vi "New Round.vi"(8 "error in (no error)":errorcluster, 10 "Move Count":i32, 11 "Grid in":T1) -> (0 "error out":errorcluster, 3 "Grid out":T1)   [LabVIEW 2015, in "TeamEffort.lvclass"]
uses:
  TeamEffort.lvclass
  Grid Cluster.ctl
  Player Cluster.ctl
  Square/Square.lvclass
  Team Move Input.ctl
  Type Defs/Action Enum.ctl
  Team Move Output.ctl
  Type Defs/Direction Enum.ctl
  Type Defs/SB Type Defs.lvlib
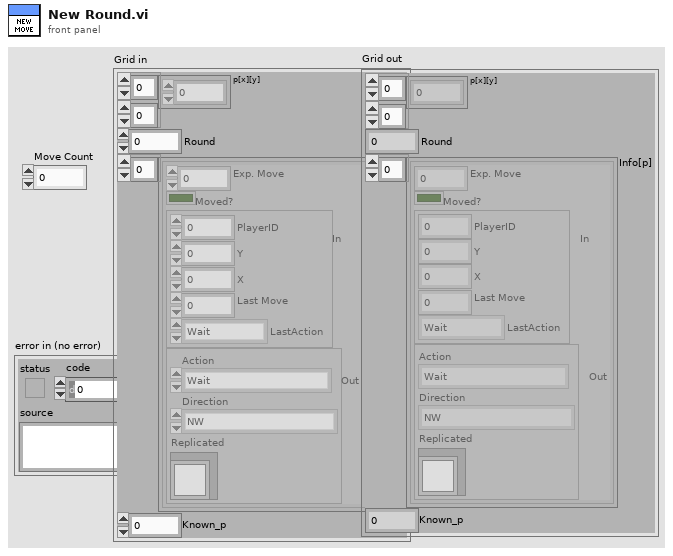
[diagram p1: front panel]
types:
  T1 = typedef "TeamEffort.lvclass/Grid Cluster.ctl" = cluster{"p[x][y]":i32[][], "Round":i32, "Info[p]":T2[], "Known_p":i32}
  T2 = typedef "TeamEffort.lvclass/Player Cluster.ctl" = cluster{"Exp. Move":i32, "Moved?":bool, "In":T3, "Out":T5}
  T3 = typedef "TeamEffort.lvclass/Team Move Input.ctl" = cluster{"PlayerID":i32, "Y":i32, "X":i32, "Last Move":i32, "LastAction":T4}
  T4 = typedef "SB Type Defs.lvlib/Action Enum.ctl" = enum16{"Wait", "Move", "Attack", "Replicate"}
  T5 = typedef "TeamEffort.lvclass/Team Move Output.ctl" = cluster{"Action":T4, "Direction":T6, "Replicated":refnum<class "Square.lvclass">}
  T6 = typedef "SB Type Defs.lvlib/Direction Enum.ctl" = enum16{"NW", "N", "NE", "E", "SE", "S", "SW", "W"}
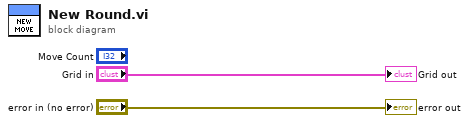
[diagram p0: block diagram]
diagram:
  "error out" <- "error in (no error)"
  "Grid out" <- "Grid in"
